vi "Update Test Sector Array FG.vi"(8 "Sector":u8, 9 "Y Pos":u16, 10 "X Pos":u16, 11 "Operation":enum16{"Read", "Write"}(ring)) -> (2 "[Test Sectors]":T1[](array[typedef]))   [LabVIEW 2013]
uses:
  Test Sector Cluster.ctl
panel:
  in  "Test Sector":T1
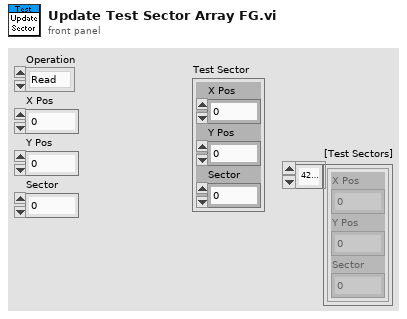
[diagram p1: front panel]
types:
  T1 = typedef "Test Sector Cluster.ctl" = cluster{"X Pos":u16, "Y Pos":u16, "Sector":u8}
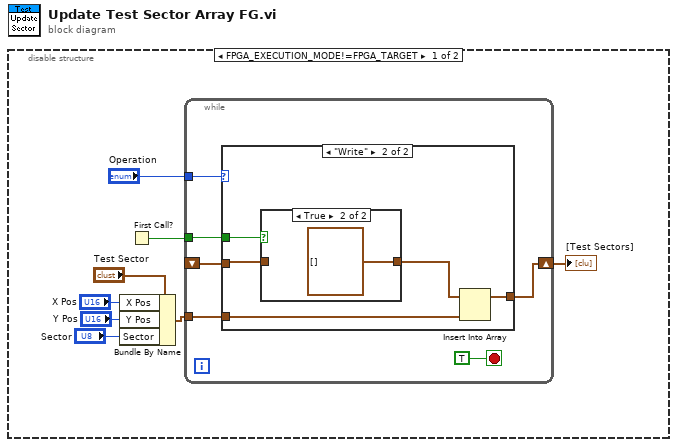
[diagram p0: block diagram]
diagram:
  n1 = disable-structure shown="FPGA_EXECUTION_MODE!=FPGA_TARGET" {
    frame condition #0 (active) {
      n2 = Bundle By Name(cluster="Test Sector", "X Pos"="X Pos", "Y Pos"="Y Pos", "Sector"="Sector") -> (w4:T1)
      n3 = First Call?() -> (First Call?: T/F=w8:bool)
      n4 = while {
        shift-right: [w11] -> w6
        shift-left: _ -> [w10]
        tunnel: w8 -> [w13]
        tunnel: w4 -> [w12]
        tunnel: "Operation" -> [w9]
        stop <- TRUE stop-if-true
        n5 = case shown="\"Write\"" w9 {
          tunnel: w13 -> [_ w20]
          tunnel: w12 -> [_ w19]
          tunnel: [w15 w18] -> w11
          tunnel: w10 -> [w15 w17]
          frame "Read" {
          }
          frame "Write" {
            n6 = case shown="True" w20 {
              tunnel: [w21 T1[] [] ("[Test Sectors]")] -> w16
              tunnel: w17 -> [w21 _]
              frame False {
              }
              frame True {
              }
            }
            n7 = Insert Into Array(array=w16, new element=w19) -> (w18:T1[])  [unwired: 1 in]
          }
        }
      }
      "[Test Sectors]" <- w6
    }
    frame condition #1 {
    }
  }
